vi "DAQmx Create Channel (AI-Strain-Strain Gage).vi"(0 "task in":refnum<k21>, 1 "maximum value":dbl=0.001 format="%0.7f", 2 "minimum value":dbl=-0.001 format="%0.7f", 5 "physical channels":tag, 7 "name to assign":string, 9 "units":i32(ring)=10299 items=["Strain"=10299, "From Custom Scale"=10065], 11 "error in":errorcluster, 12 "custom scale name":tag, 13 "bridge information":T1={"strain configuration"=10183, "lead wire resistance"=0.0, "initial bridge voltage"=0.0, "voltage excitation source"=10200, "voltage excitation value"=2.5} {"initial bridge voltage" format="%0.2f"; "voltage excitation source" items=["Internal"=10200, "External"=10167, "None"=10230]; "voltage excitation value" format="%0.2f"; "lead wire resistance" format="%0.2f"; "strain configuration" items=["Full Bridge I"=10183, "Full Bridge II"=10184, "Full Bridge III"=10185, "Half Bridge I"=10188, "Half Bridge II"=10189, "Quarter Bridge I"=10271, "Quarter Bridge II"=10272]}, 14 "strain gage information":T2={"gage factor"=2.0, "nominal gage resistance"=350.0, "poisson ratio"=0.3} {"poisson ratio" format="%0.2f"; "nominal gage resistance" format="%0.2f"; "gage factor" format="%0.2f"}) -> (4 "task out":refnum<k21>, 15 "error out":errorcluster)   [LabVIEW 2013]
doc: "Creates channel(s) to measure strain."
uses:
  <resource>/objmgr/daqmx.rc
panel:
  # "input limits"
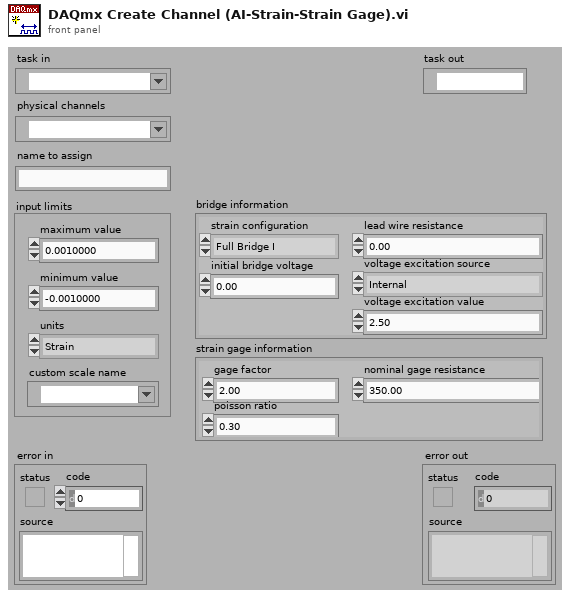
[diagram p1: front panel]
types:
  T1 = cluster{"strain configuration":i32, "lead wire resistance":dbl, "initial bridge voltage":dbl, "voltage excitation source":i32, "voltage excitation value":dbl}
  T2 = cluster{"gage factor":dbl, "nominal gage resistance":dbl, "poisson ratio":dbl}
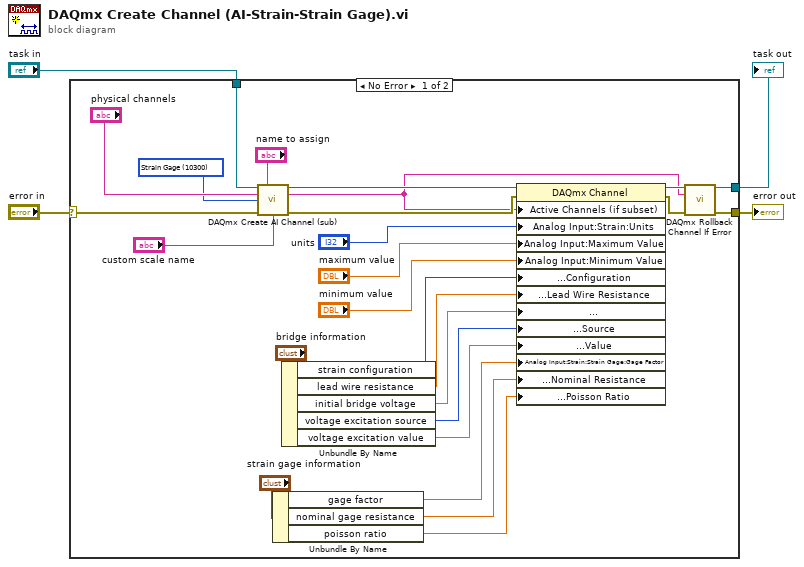
[diagram p0: block diagram]
diagram:
  n1 = case shown="No Error" "error in" {
    selector: "error in" -> [w29 w31]
    tunnel: [w8 w31] -> w4
    tunnel: "task in" -> [w30 w32]
    tunnel: [w7 w32] -> w1
    frame No Error {
      w21 = 10300 items=["Voltage"=10322, "Current"=10134, "More:Voltage:Custom with Excitation"=10323, "More:Current:Custom with Excitation"=10136, "Frequency"=10181, "Period"=10257, "Resistance"=10278, "Temperature:Thermocouple"=10303, "Temperature:Thermistor"=10302, "Temperature:RTD"=10301, "Temperature:Built-in Sensor"=10311, "Strain Gage"=10300] ("measurement type")
      n2 = call "DAQmx Create AI Channel (sub).vi"("task in"=w30, "virtual channel name"="name to assign", "physical channel name"="physical channels", "measurement type"=w21, "error in"=w29, "custom scale"="custom scale name") -> ("task out"=w26:refnum<k21>, "channel names"=w5:string, "error out"=w20:errorcluster)  [unwired: 1 in, 6 out]
      n3 = Unbundle By Name("strain gage information") -> ("gage factor"=w12:dbl, "nominal gage resistance"=w11:dbl, "poisson ratio"=w10:dbl)
      n4 = Unbundle By Name("bridge information") -> ("strain configuration"=w17:i32, "lead wire resistance"=w16:dbl, "initial bridge voltage"=w15:dbl, "voltage excitation source"=w14:i32, "voltage excitation value"=w13:dbl)
      n5 = property class="DAQmx Channel"(reference=w26, error in=w20, "Active Channels (if subset)"=w5, "Analog Input:Strain:Units"="units", "Analog Input:Maximum Value"="maximum value", "Analog Input:Minimum Value"="minimum value", "Analog Input:Strain:Strain Gage:Configuration"=w17, "Analog Input:General Properties:Signal Conditioning:Lead Wire Resistance"=w16, "Analog Input:General Properties:Signal Conditioning:Bridge:Initial Bridge Voltage"=w15, "Analog Input:General Properties:Signal Conditioning:Excitation:Source"=w14, "Analog Input:General Properties:Signal Conditioning:Excitation:Value"=w13, "Analog Input:Strain:Strain Gage:Gage Factor"=w12, "Analog Input:General Properties:Signal Conditioning:Bridge:Nominal Resistance"=w11, "Analog Input:Strain:Strain Gage:Poisson Ratio"=w10) -> (reference out=w9:refnum<k21>, error out=w6:errorcluster)
      n6 = call "DAQmx Rollback Channel If Error.vi"("task in"=w9, "channel names"=w5, "error in"=w6) -> ("task out"=w7:refnum<k21>, "error out"=w8:errorcluster)  [unwired: 11 out]
    }
    frame Error {
    }
  }
  "error out" <- w4
  "task out" <- w1
